vi "REPORT_OPRTN_add_record_when_reshaping.vi"(7 "no_of_dynamic_columns":i32, 9 "records_from_SQL":string[](array[string]), 10 "last_row_in":i32, 11 "records_to_display_in":string[][](array[string])) -> (2 "last_row_out":i32, 3 "records_to_display_out":string[][](array[string]))   [LabVIEW 2019]
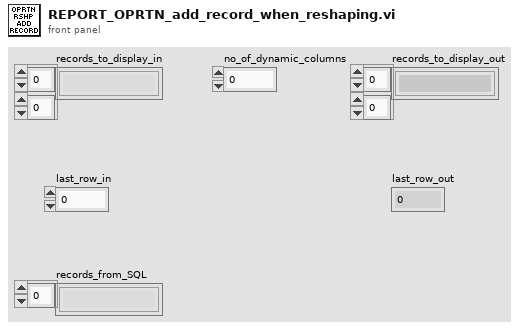
[diagram p1: front panel]
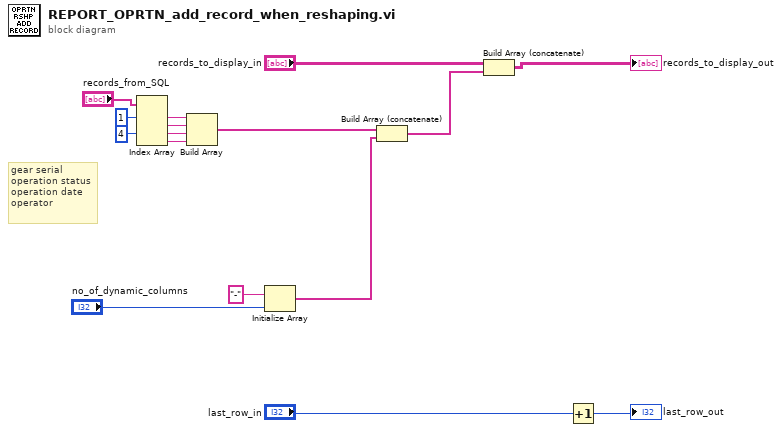
[diagram p0: block diagram]
diagram:
  # "gear serial\noperation status\noperation date\noperator"
  n1 = Index Array(array="records_from_SQL", index #1=1 ("index"), index #3=4 ("index")) -> (element #1=w8:string, element #2=w9:string, element #3=w10:string, element #4=w11:string)  [unwired: 2 in]
  n2 = Build Array(w8, w9, w10, w11) -> (w2:string[])
  n3 = Initialize Array("-", "no_of_dynamic_columns") -> (w1:string[])
  n4 = Build Array (concatenate)(w2, w1) -> (w3:string[])
  n5 = Build Array (concatenate)("records_to_display_in", w3) -> (→"records_to_display_out":string[][])
  n6 = Increment(x="last_row_in") -> (x+1=→"last_row_out":i32)
